vi "Generate Waveforms.vi"(1 "Aggregate Sound.lvclass":refnum<class "Aggregate Sound.lvclass">) -> (0 "Waveforms":waveform(dbl)[](array[waveform]))   [LabVIEW 2010, in "Aggregate Sound.lvclass"]
uses:
  Aggregate Sound.lvclass
  Aggregate Sound.lvclass/Aggregate Sound.ctl
  <vilib>/Waveform/WDTOps.llb/WDT Align Waveform Timestamps DBL.vi
  Sound/Sound.lvclass
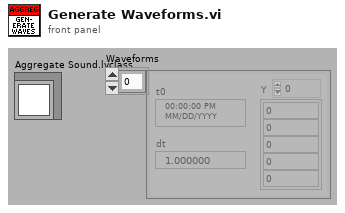
[diagram p1: front panel]
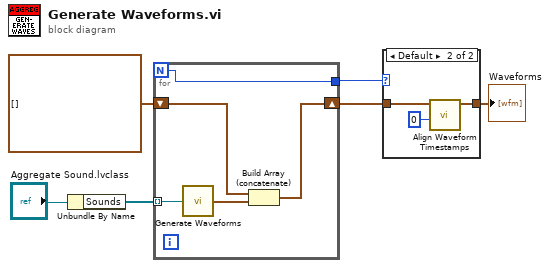
[diagram p0: block diagram]
diagram:
  n1 = Unbundle By Name("Aggregate Sound.lvclass") -> ("Sounds"=w5:refnum<class "Sound.lvclass">[])
  n2 = for {
    N -> [w7]
    tunnel: w5 -> [w11] mode=indexing
    shift-right: [w9] -> w3
    shift-left: waveform(dbl)[] [] ("Waveforms") -> [w10]
    tunnel: [w7] -> w1
    n3 = call-dynamic "Generate Waveforms.vi"("Sound.lvclass"=w11) -> ("Waveforms"=w8:waveform(dbl)[])
    n4 = Build Array (concatenate)(w10, w8) -> (w9:waveform(dbl)[])
  }
  n5 = case shown="Default" w1 {
    tunnel: w3 -> [w12 w14]
    tunnel: [w12 w13] -> w2
    frame 0 {
    }
    frame Default {
      n6 = call-poly <vilib>:"Align Waveform Timestamps.vi"("index"=0, "waveforms in"=w14) -> ("waveforms out"=w13:waveform(dbl)[])  [unwired: 8 in, 1 out]
    }
  }
  "Waveforms" <- w2
